vi "Set Instrument Addon Name.vi"(8 "error in (no error)":errorcluster, 10 "name":string, 11 "instrument addon refnum in":T1 format="%.0x") -> (0 "error out":errorcluster, 3 "instrument addon refnum out":T1=18446744073709551615 format="%.0x")   [LabVIEW 2018, in "Instrument Addon Scripting API.lvlib"]
doc: "Sets the Instrument Addon Custom Device to the specified name."
uses:
  Instrument Addon Scripting API.lvlib
  <vilib>/NI Veristand/Custom Device API/Custom Device Item Ref.ctl
  <vilib>/NI Veristand/Custom Device API/Custom Device API.lvlib
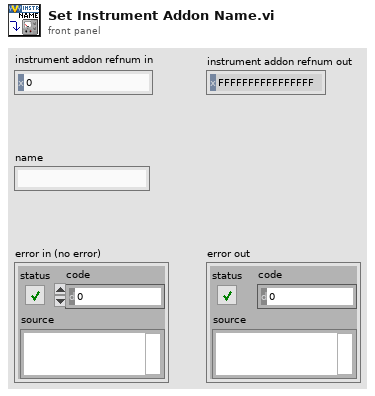
[diagram p1: front panel]
types:
  T1 = typedef "Custom Device API.lvlib/Custom Device Item Ref.ctl" = u64
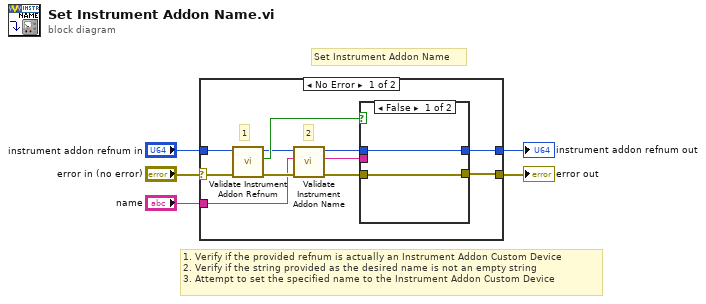
[diagram p0: block diagram]
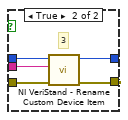
[diagram p2: hidden frame]
diagram:
  # "1. Verify if the provided refnum is actually an Instrument Addon Custom Device\n2. Verify if the string provided as the desired name is not an empty string\n3. Attempt to set the specified name to the Instrument Addon Custom Device"
  # "Set Instrument Addon Name"
  n1 = case shown="No Error" "error in (no error)" {
    selector: "error in (no error)" -> [w16 w25]
    tunnel: "instrument addon refnum in" -> [w15 w24]
    tunnel: [w13 w25] -> w4
    tunnel: [w12 w24] -> w2
    tunnel: "name" -> [w9 _]
    frame No Error {
      # "2"
      # "1"
      n2 = call "Validate Instrument Addon Refnum.vi"("Error In"=w16, "Refnum In"=w15) -> ("Error Out"=w10:errorcluster, "Is Instrument Addon?"=w14:bool, "Refnum Out"=w11:T1)  [unwired: 7 in]
      n3 = call "Validate Instrument Addon Name.vi"("Error In"=w10, "Name In"=w9, "Instrument Addon Refnum In"=w11) -> ("Error Out"=w7:errorcluster, "Name Out"=w8:string, "Instrument Addon Refnum Out"=w6:T1)  [unwired: 6 in]
      n4 = case shown="False" w14 {
        tunnel: [w17 w23] -> w13
        tunnel: [w18 w22] -> w12
        tunnel: w8 -> [_ w21]
        tunnel: w7 -> [w17 w20]
        tunnel: w6 -> [w18 w19]
        frame False {
        }
        frame True {
          # "3"
          n5 = call <vilib>:"NI VeriStand - Rename Custom Device Item.vi"("error in (no error)"=w20, "New Name"=w21, "Item Ref in"=w19) -> ("error out"=w23:errorcluster, "Item Ref out"=w22:T1)  [unwired: 6 in, 1 out]
        }
      }
    }
    frame Error {
    }
  }
  "error out" <- w4
  "instrument addon refnum out" <- w2
